vi "Read DAQ.Config.vi"(8 "error in (no error)":errorcluster, 11 "DAQ in":refnum<class "DAQ.lvclass">) -> (0 "error out":errorcluster, 2 "Configuration":T1={"Channels"="", "DAQType"=enum."AI", "minimum value"=-5.0, "maximum value"=5.0, "sampling info"={"Fs"=0.0, "#s"=0.0}, "SamplingMode"=enum."Continuous"} {"maximum value" format="%0.2f"; "minimum value" format="%0.2f"}, 3 "DAQ out":refnum<class "DAQ.lvclass">)   [LabVIEW 2016, in "DAQ.lvclass"]
uses:
  DAQ.lvclass
  Typedefs/DAQ.Config.ctl
  Typedefs/PrivateEvents--DAQ.AI.Channels.ctl
  Typedefs/DAQType.ctl
  Typedefs/SamplingInfo.ctl
  Typedefs/SamplingMode.ctl
  DAQ.lvclass/DAQ.ctl
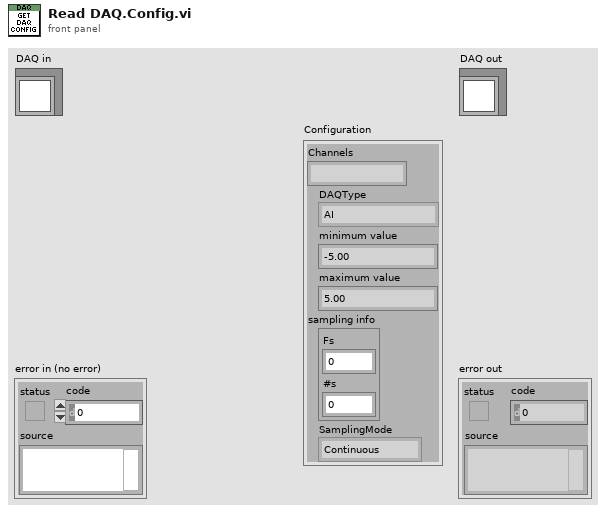
[diagram p1: front panel]
types:
  T1 = typedef "DAQ.lvclass/DAQ.Config.ctl" = cluster{"Channels":T2, "DAQType":T3, "minimum value":dbl, "maximum value":dbl, "sampling info":T4, "SamplingMode":T5}
  T2 = typedef "PrivateEvents--DAQ.AI.Channels.ctl" = string
  T3 = typedef "DAQ.lvclass/DAQType.ctl" = enum16{"AI", "AO"}
  T4 = typedef "DAQ.lvclass/SamplingInfo.ctl" = cluster{"Fs":dbl, "#s":dbl}
  T5 = typedef "DAQ.lvclass/SamplingMode.ctl" = enum16{"Continuous", "Finite"}
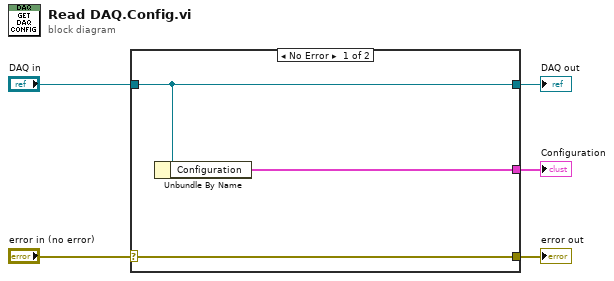
[diagram p0: block diagram]
diagram:
  n1 = case shown="No Error" "error in (no error)" {
    selector: "error in (no error)" -> [w8 w9]
    tunnel: [w8 w9] -> w4
    tunnel: [w7 w10] -> w2
    tunnel: "DAQ in" -> [w7 w10]
    tunnel: [w6 _] -> w1
    frame No Error {
      n2 = Unbundle By Name(w7) -> ("Configuration"=w6:T1)
    }
    frame Error {
    }
  }
  "error out" <- w4
  "DAQ out" <- w2
  "Configuration" <- w1
